vi "INTELLIFAUCET Start Stop.vi"(7 "Start?":bool, 8 "error in (no error)":errorcluster, 11 "VISA Refnum in":refnum<visa-resource-name>) -> (0 "error out":errorcluster, 3 "VISA Refnum out":refnum<visa-resource-name>)   [LabVIEW 2023]
uses:
  Type Definitions/HEWH Normally Open Valve Control.ctl
  MW100/Type Definitions/HEWH MW100 Channel Numbers.ctl
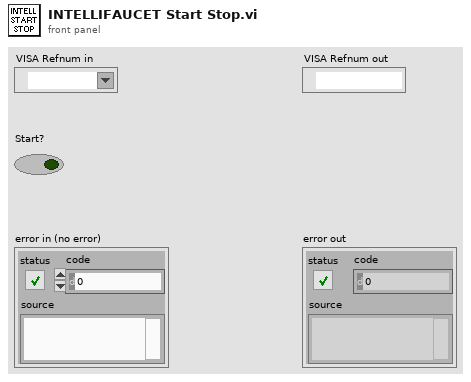
[diagram p1: front panel]
types:
  T1 = typedef "HEWH Normally Open Valve Control.ctl" = string
  T2 = typedef "HEWH MW100 Channel Numbers.ctl" = string
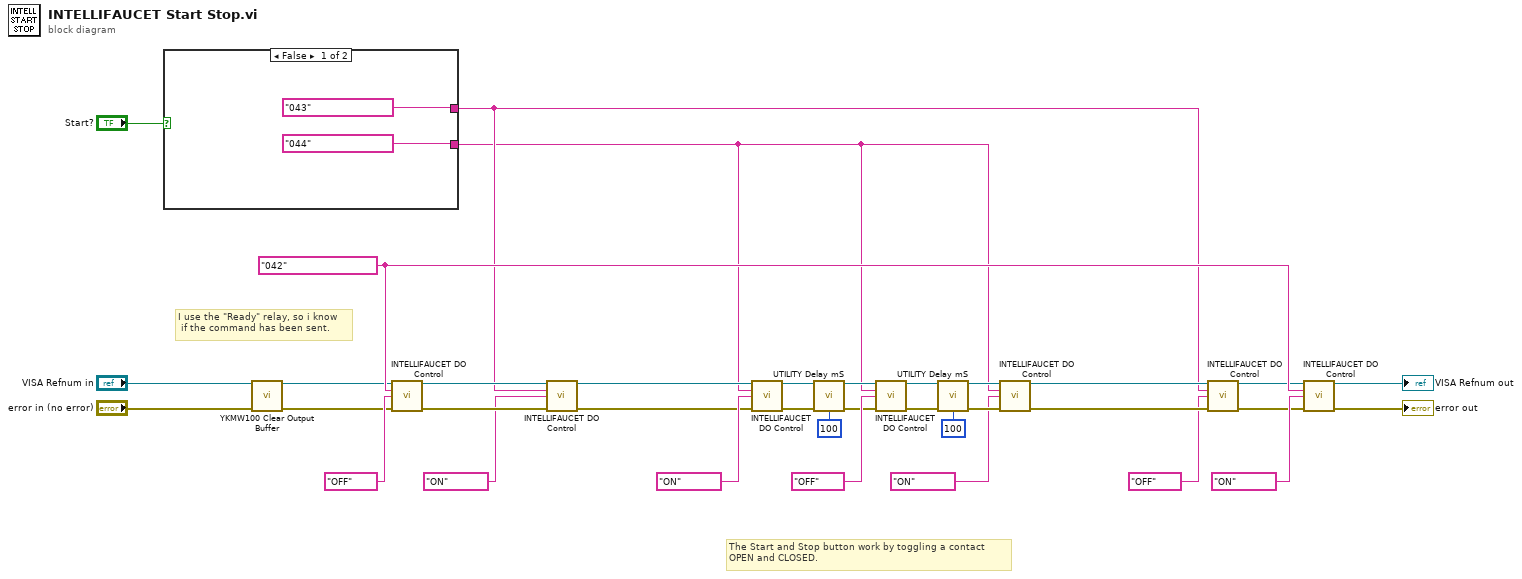
[diagram p0: block diagram]
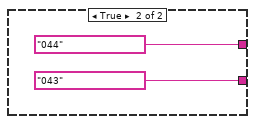
[diagram p2: hidden frame]
diagram:
  w32 = T2 "042" ("HEWH MW100 Channel Numbers")
  # "I use the \"Ready\" relay, so i know\n if the command has been sent."
  # "The Start and Stop button work by toggling a contact\nOPEN and CLOSED."
  n1 = case shown="False" "Start?" {
    tunnel: [T2 "043" ("HEWH MW100 Channel Numbers") T2 "044" ("HEWH MW100 Channel Numbers")] -> w11
    tunnel: [T2 "044" ("HEWH MW100 Channel Numbers") T2 "043" ("HEWH MW100 Channel Numbers")] -> w2
    frame False {
    }
    frame True {
    }
  }
  n2 = call "YKMW100 Clear Output Buffer.vi"("VISA session"="VISA Refnum in", "error in (no error)"="error in (no error)") -> ("dup VISA session"=w24:refnum<visa-resource-name>, "error out"=w23:errorcluster)  [unwired: 12 in]
  n3 = call "INTELLIFAUCET DO Control.vi"("VISA session"=w24, "HEWH MW100 Channel Numbers"=w32, "Normally Open"=T1 "OFF", "Error In"=w23) -> ("dup VISA session"=w25:refnum<visa-resource-name>, "error out"=w26:errorcluster)  [unwired: 10 in]
  n4 = call "INTELLIFAUCET DO Control.vi"("VISA session"=w25, "HEWH MW100 Channel Numbers"=w11, "Normally Open"=T1 "ON", "Error In"=w26) -> ("dup VISA session"=w10:refnum<visa-resource-name>, "error out"=w9:errorcluster)  [unwired: 10 in]
  n5 = call "INTELLIFAUCET DO Control.vi"("VISA session"=w10, "HEWH MW100 Channel Numbers"=w2, "Normally Open"=T1 "ON" ("Normally Open Valve"), "Error In"=w9) -> ("dup VISA session"=w4:refnum<visa-resource-name>, "error out"=w6:errorcluster)  [unwired: 10 in]
  n6 = call "UTILITY Delay mS.vi"("Error In"=w6, "milliseconds to wait"=u32 100) -> ("Error Out"=w7:errorcluster)  [unwired: 13 in]
  n7 = call "INTELLIFAUCET DO Control.vi"("VISA session"=w4, "HEWH MW100 Channel Numbers"=w2, "Normally Open"=T1 "OFF", "Error In"=w7) -> ("dup VISA session"=w17:refnum<visa-resource-name>, "error out"=w21:errorcluster)  [unwired: 10 in]
  n8 = call "UTILITY Delay mS.vi"("Error In"=w21, "milliseconds to wait"=u32 100) -> ("Error Out"=w22:errorcluster)  [unwired: 13 in]
  n9 = call "INTELLIFAUCET DO Control.vi"("VISA session"=w17, "HEWH MW100 Channel Numbers"=w2, "Normally Open"=T1 "ON", "Error In"=w22) -> ("dup VISA session"=w18:refnum<visa-resource-name>, "error out"=w16:errorcluster)  [unwired: 10 in]
  n10 = call "INTELLIFAUCET DO Control.vi"("VISA session"=w18, "HEWH MW100 Channel Numbers"=w11, "Normally Open"=T1 "OFF" ("Normally Open Valve"), "Error In"=w16) -> ("dup VISA session"=w28:refnum<visa-resource-name>, "error out"=w30:errorcluster)  [unwired: 10 in]
  n11 = call "INTELLIFAUCET DO Control.vi"("VISA session"=w28, "HEWH MW100 Channel Numbers"=w32, "Normally Open"=T1 "ON", "Error In"=w30) -> ("dup VISA session"=→"VISA Refnum out":refnum<visa-resource-name>, "error out"=→"error out":errorcluster)  [unwired: 10 in]
